vi "Array2String.vi"(5 "Size":u8, 7 "Hex Array":u8[](array[numeric])) -> (8 "HEX String":string)   [LabVIEW 2017]
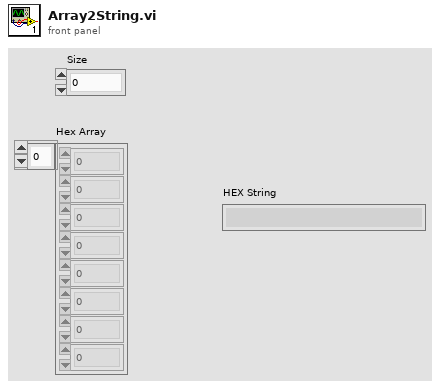
[diagram p1: front panel]
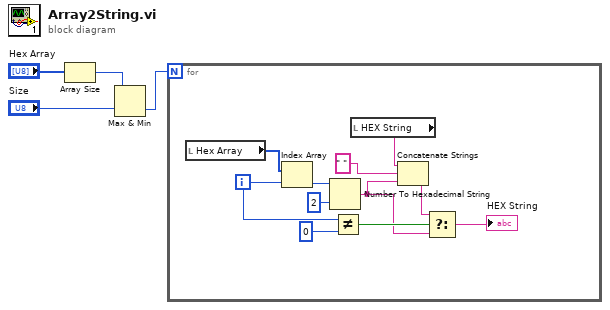
[diagram p0: block diagram]
diagram:
  n1 = Array Size(array="Hex Array") -> (size(s)=w3:i32)
  n2 = Max & Min(x=w3, y="Size") -> (min(x,y)=w1:i32)  [unwired: 1 out]
  n3 = for {
    N: w1 -> [_]
    i -> [w12]
    n4 = local read "Hex Array"() -> (w15:u8[])
    n5 = Index Array(array=w15, index=w12) -> (element=w14:u8)
    n6 = Number To Hexadecimal String(1:i16 2 ("宽度(-)"), 2:w14) -> (0:w5:string)
    n7 = Not Equal?(x=w12, y=0) -> (x != y?=w10:bool)
    n8 = local read "HEX String"() -> (w9:string)
    n9 = Concatenate Strings(w9, " " ("字符串"), w5) -> (w7:string)
    n10 = Select(t=w7, s=w10, f=w5) -> (s? t:f=→"HEX String":string)
  }
